vi "for_v0_v5.vi"() -> ()   [LabVIEW 2010]
panel:
  in  "Stop":bool
  in  "Nr_max":u8(slide)=60 scale=0.0..255.0
  out "Numeric":dbl=48.0
  out "Array":bool[](array[boolean])=[FALSE, FALSE, TRUE, TRUE, FALSE, FALSE, FALSE, FALSE]
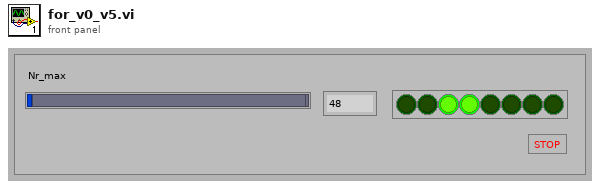
[diagram p1: front panel]
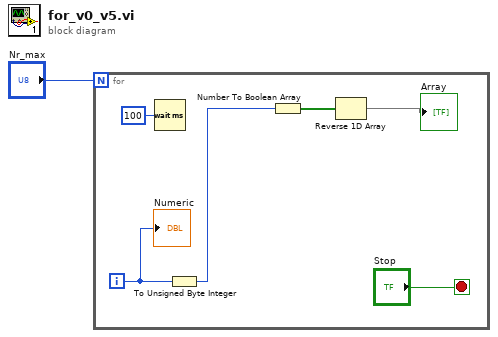
[diagram p0: block diagram]
diagram:
  n1 = for {
    N: "Nr_max" -> [_]
    i -> [w3]
    stop <- "Stop" stop-if-true
    n2 = Wait (ms)(milliseconds to wait=u32 100) -> ()  [unwired: 1 out]
    n3 = To Unsigned Byte Integer(number=w3) -> (unsigned 8bit integer=w4:u8)
    n4 = Number To Boolean Array(number=w4) -> (Boolean array=w7:bool[])
    n5 = Reverse 1D Array(array=w7) -> (reversed array=→"Array":bool[])
    "Numeric" <- w3
  }
